vi "Lockin_Example_IV_Curves.vi"() -> ()   [LabVIEW 2013]
panel:
  out "2 terminal":cluster{"Y":dbl[], "Y":dbl[]}(graph)
  out "4 terminal":cluster{"Y":dbl[], "Y":dbl[]}(graph)
  in  "step":dbl=0.025
  in  "end":dbl=0.1
  in  "start":dbl
  in  "Channels: AO":T1={"AO amp (V)"=[0.1, 0.2, 0.0, 0.0, 0.0, 0.0, 0.0, 0.0], "AO DC (V)"=[0.0, 0.0, 0.0, 0.0, 0.0, 0.0, 0.0, 0.0], "AO f (Hz)"=[1.0, 1.0, 1.0, 1.0, 1.0, 1.0, 1.0, 1.0], "AO phi (deg)"=[0.0, 0.0, 0.0, 0.0, 0.0, 0.0, 0.0, 0.0], "function"=[enum."Triangle Wave", enum."Triangle Wave", enum."Sine Wave", enum."Sine Wave", enum."Sine Wave", enum."Sine Wave", enum."Sine Wave", enum."Sine Wave"]} {"AO DC (V)" format="%#_6p"; "AO amp (V)" format="%#_6p"}
  # "Lockin Example: IV Curves\nMake Sure Lockin Program is running!"
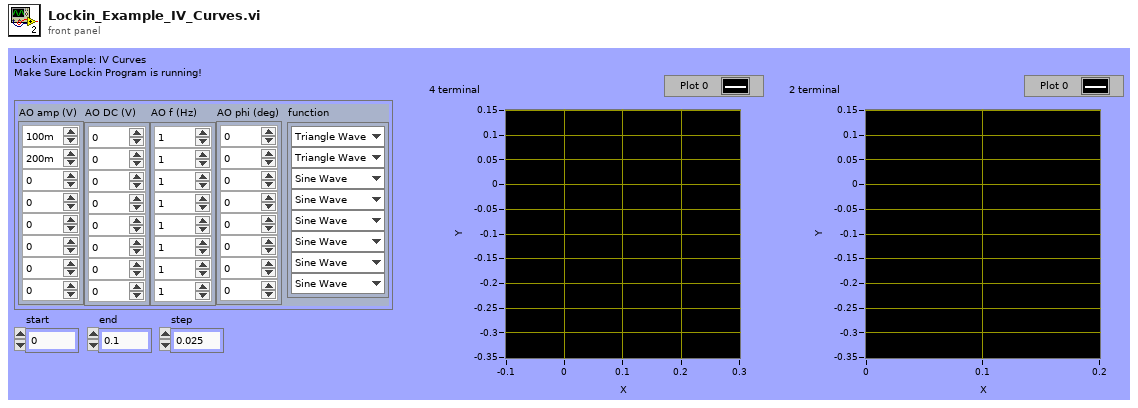
[diagram p1: front panel]
types:
  T1 = cluster{"AO amp (V)":dbl[], "AO DC (V)":dbl[], "AO f (Hz)":dbl[], "AO phi (deg)":dbl[], "function":enum16{"Sine Wave", "Triangle Wave", "Square Wave", "Sawtooth Wave"}[]}
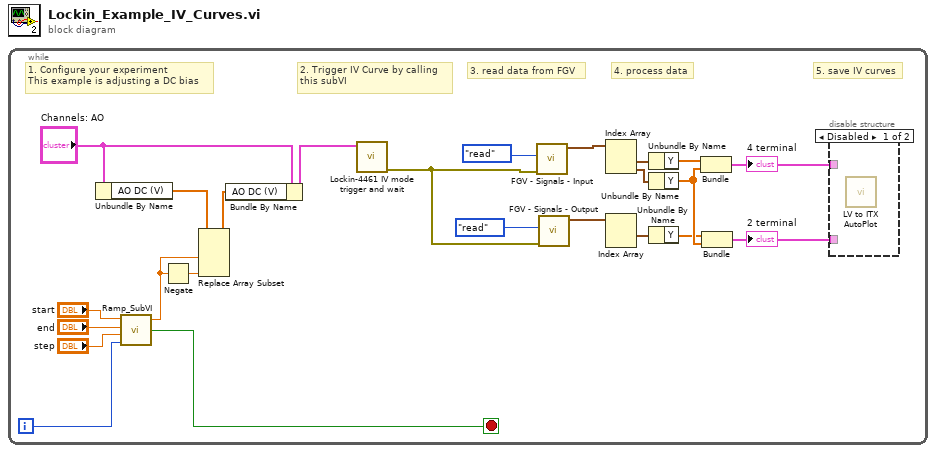
[diagram p0: block diagram]
diagram:
  n1 = while {
    i -> [w15]
    stop <- w24 stop-if-true
    # "5. save IV curves"
    # "4. process data"
    # "3. read data from FGV"
    # "1. Configure your experiment\nThis example is adjusting a DC bias"
    # "2. Trigger IV Curve by calling\nthis subVI"
    n2 = Unbundle By Name("Channels: AO") -> ("AO DC (V)"=w21:dbl[])
    n3 = call <userlib>:"Ramp_SubVI.vi"("index"=w15, "step"="step", "end"="end", "start"="start") -> ("Stop?"=w24:bool, "Numeric"=w19:dbl)  [unwired: 1 in]
    n4 = Negate(x=w19) -> (-x=w17:dbl)
    n5 = Replace Array Subset(array=w21, new element #1=w19, new element #2=w17) -> (w20:dbl[])  [unwired: 2 in]
    n6 = Bundle By Name(cluster="Channels: AO", "AO DC (V)"=w20) -> (w23:T1)
    n7 = call "Lockin-4461 IV mode trigger and wait.vi"("Channels: AO"=w23) -> ("error out"=w3:errorcluster)  [unwired: 10 in]
    n8 = call "FGV - Signals - Input.vi"("error in"=w3, "Function"=enum16{"write", "read"}."read") -> ("input signal"=w4:waveform(dbl)[])  [unwired: 4 in, 1 out]
    n9 = call "FGV - Signals - Output.vi"("error in"=w3, "Function"=enum16{"write", "read"}."read") -> ("input signal"=w2:waveform(dbl)[])  [unwired: 4 in, 1 out]
    n10 = Index Array(array=w4) -> (element #1=w13:waveform(dbl), element #2=w11:waveform(dbl))  [unwired: 2 in]
    n11 = Index Array(array=w2) -> (element #1=w10:waveform(dbl))  [unwired: 2 in, 1 out]
    n12 = Unbundle By Name(w13) -> ("Y"=w12:dbl[])
    n13 = Unbundle By Name(w11) -> ("Y"=w9:dbl[])
    n14 = Unbundle By Name(w10) -> ("Y"=w8:dbl[])
    n15 = Bundle("Y"=w12, "Y"=w9) -> (w7:cluster{"Y":dbl[], "Y":dbl[]})  [unwired: 1 in]
    "4 terminal" <- w7
    n16 = Bundle("Y"=w8, "Y"=w9) -> (w6:cluster{"Y":dbl[], "Y":dbl[]})  [unwired: 1 in]
    "2 terminal" <- w6
    n17 = disable-structure shown="Disabled" {
      disable-tunnel: w7 -> [_ _]
      disable-tunnel: w6 -> [_ _]
      frame Disabled {
        n18 = call <userlib>:"LV to ITX AutoPlot.vi"() -> ()  [unwired: 15 in, 1 out]
      }
      frame Enabled {
      }
    }
  }
